vi "Configure Signal (Common).vi"(0 "niUsrpRio Session":T3={"Global Settings Register Bus"=refnum, "Radio 0 Settings Register Bus"=refnum, "Rx NI-USRP session"="", "Tx NI-USRP session"="", "FPGA Interface"=refnum, "RIO Interface Number"=0, "EEPROM Header"={"Checksum"=0, "Product Code"=0, "Hardware Current Version"=0, "Hardware Oldest Compatible Version"=0, "EEPROM Map Current Version"=0, "EEPROM Map Oldest Compatible Version"=0, "User Password"="", "Pointer to Factory Header"=0, "Pointer to User Header"=0, "Recommended Interval"=0, "Number of Reserved Bytes"=9, "Number of Daughterboards"=0, "Daughterboard IDs"=[], "Daughterboard Serial Numbers"=[]}, "Device Data Header"={"Checksum"=0, "Number of Channels"=0, "Number of Gain Settings"=[], "Pointer to Characterization Data"=[], "Number of Reserved Bytes"=27, "Number of Frequencies"=[]}, "EEPROM Characterization Header"={"Checksum"=0, "Date"=timestamp(0 s since 1904-01-01), "Temperature"=0.0, "Misc. Info"="", "Pointer to Device Data Header"=0, "Number of Reserved Bytes"=28}, "Characterization Data"=[], "Characterization Data Valid?"=FALSE, "Radio 1 Settings Register Bus"=refnum, "Radio Settings Bus Semaphore"=refnum} {"Characterization Data"."Frequencies [Hz]" format="%#_6p"; "EEPROM Characterization Header"."Pointer to Device Data Header" format="%x"; "EEPROM Characterization Header"."Checksum" format="%x"; "Device Data Header"."Pointer to Characterization Data" format="%x"; "Device Data Header"."Checksum" format="%x"; "EEPROM Header"."Pointer to User Header" format="%x"; "EEPROM Header"."Pointer to Factory Header" format="%x"; "EEPROM Header"."Product Code" format="%x"; "EEPROM Header"."Checksum" format="%x"}, 1 "scope":string(combo)="rx", 2 "Correct Impairments?":bool=TRUE, 5 "signal parameters":T2={"gain/level"=0.0, "sample rate [S/s]"=10000000.0, "frequency [Hz]"=2450000000.0, "LO frequency [Hz]"=-1.0, "active antenna"="RX1"} {"LO frequency [Hz]" format="%#.3pHz"; "frequency [Hz]" format="%#.3pHz"; "sample rate [S/s]" min=1.0 max=250000000.0 format="%#.3pS/s"}, 7 "Configure Signal Mode":T1, 11 "error in":errorcluster) -> (4 "niUsrpRio Session (out)":T3={"Global Settings Register Bus"=refnum, "Radio 0 Settings Register Bus"=refnum, "Rx NI-USRP session"="", "Tx NI-USRP session"="", "FPGA Interface"=refnum, "RIO Interface Number"=0, "EEPROM Header"={"Checksum"=0, "Product Code"=0, "Hardware Current Version"=0, "Hardware Oldest Compatible Version"=0, "EEPROM Map Current Version"=0, "EEPROM Map Oldest Compatible Version"=0, "User Password"="", "Pointer to Factory Header"=0, "Pointer to User Header"=0, "Recommended Interval"=0, "Number of Reserved Bytes"=9, "Number of Daughterboards"=0, "Daughterboard IDs"=[], "Daughterboard Serial Numbers"=[]}, "Device Data Header"={"Checksum"=0, "Number of Channels"=0, "Number of Gain Settings"=[], "Pointer to Characterization Data"=[], "Number of Reserved Bytes"=27, "Number of Frequencies"=[]}, "EEPROM Characterization Header"={"Checksum"=0, "Date"=timestamp(0 s since 1904-01-01), "Temperature"=0.0, "Misc. Info"="", "Pointer to Device Data Header"=0, "Number of Reserved Bytes"=28}, "Characterization Data"=[], "Characterization Data Valid?"=FALSE, "Radio 1 Settings Register Bus"=refnum, "Radio Settings Bus Semaphore"=refnum} {"Characterization Data"."Frequencies [Hz]" format="%#_6p"; "EEPROM Characterization Header"."Pointer to Device Data Header" format="%x"; "EEPROM Characterization Header"."Checksum" format="%x"; "Device Data Header"."Pointer to Characterization Data" format="%x"; "Device Data Header"."Checksum" format="%x"; "EEPROM Header"."Pointer to User Header" format="%x"; "EEPROM Header"."Pointer to Factory Header" format="%x"; "EEPROM Header"."Product Code" format="%x"; "EEPROM Header"."Checksum" format="%x"}, 6 "coerced signal parameters":T2={"gain/level"=0.0, "sample rate [S/s]"=10000000.0, "frequency [Hz]"=2450000000.0, "LO frequency [Hz]"=-1.0, "active antenna"="RX1"} {"LO frequency [Hz]" format="%#.3pHz"; "frequency [Hz]" format="%#.3pHz"; "sample rate [S/s]" min=1.0 max=250000000.0 format="%#.3pS/s"}, 15 "error out":errorcluster)   [LabVIEW 2013]
doc: "Configures the DSP and signal path for the channel based on the input <B>signal parameters</B>."
uses:
  <instrlib>/niUsrpRio/Config/v1/Host/Public/niUsrpRio Session.ctl
  <instrlib>/_niInstr/Register Bus/v0/Host/Public/Register Bus Session.ctl
  <instrlib>/_niInstr/Register Bus/v0/Host/Private/Session Data.ctl
  <instrlib>/niUsrpRio/Config/v1/Host/Public/EEPROM Header.ctl
  <instrlib>/niUsrpRio/Config/v1/Host/Public/EEPROM Device Data Header.ctl
  <instrlib>/niUsrpRio/Config/v1/Host/Public/EEPROM Characterization Header.ctl
  <instrlib>/niUsrpRio/Config/v1/Host/Public/Characterization Data.ctl
  <instrlib>/niUsrpRio/Config/v1/Host/Public/IQ Imbalance.ctl
  Configure Signal Parameters.ctl
  Configure Signal Mode.ctl
  <instrlib>/_niInstr/DSP/v1/Shared/Public/IQ Impairments.ctl
  Rx FPGA VI Reference.ctl
  Tx FPGA VI Reference.ctl
  <instrlib>/_niInstr/DSP/v1/Shared/Public/IQ Gain.ctl
  <vilib>/rvi/interface/common/niFpgaWaitOnOcc.vi
  <vilib>/Utility/error.llb/Error Cluster From Error Code.vi
  <vilib>/rvi/errors/niLvFpgaAdjustHostInterfaceError.vi
  <vilib>/rvi/interface/nirviReadWriteControl/nirviReadWriteControl.xnode
  <vilib>/ErrorRing/Error Ring.xnode
  NiFpgaLv.dll
  <vilib>/rvi/interface/Simulation/niFpgaSimulationCallBeginRW.vi
  <instrlib>/_niInstr/DSP/v1/Shared/niInstr DSP v1 Shared.lvlib
  <instrlib>/niUsrpRio/Config/v1/Host/niUsrpRio Config v1 Host.lvlib
  <instrlib>/_niInstr/Register Bus/v0/Host/niInstr Register Bus v0 Host.lvlib
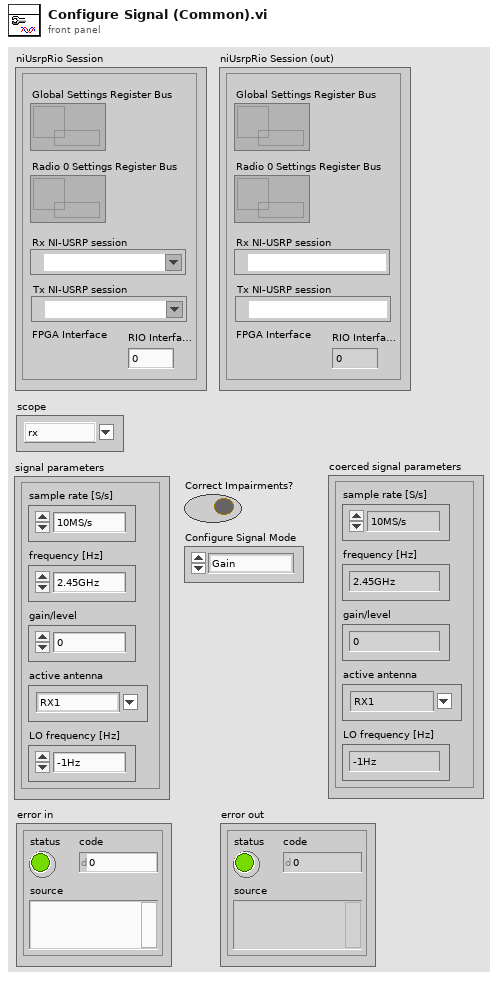
[diagram p1: front panel]
types:
  T1 = typedef "Configure Signal Mode.ctl" = enum16{"Gain", "Level"}
  T2 = typedef "Configure Signal Parameters.ctl" = cluster{"gain/level":dbl, "sample rate [S/s]":dbl, "frequency [Hz]":dbl, "LO frequency [Hz]":dbl, "active antenna":string}
  T3 = typedef "niUsrpRio Config v1 Host.lvlib/niUsrpRio Session.ctl" = cluster{"Global Settings Register Bus":T4, "Radio 0 Settings Register Bus":T4, "Rx NI-USRP session":refnum<k15>, "Tx NI-USRP session":refnum<k15>, "FPGA Interface":refnum<k20>, "RIO Interface Number":u32, "EEPROM Header":T5, "Device Data Header":T6, "EEPROM Characterization Header":T7, "Characterization Data":T8[], "Characterization Data Valid?":bool, "Radio 1 Settings Register Bus":T4, "Radio Settings Bus Semaphore":T10}
  T4 = typedef "niInstr Register Bus v0 Host.lvlib/Register Bus Session.ctl" = refnum<queue>
  T5 = typedef "niUsrpRio Config v1 Host.lvlib/EEPROM Header.ctl" = cluster{"Checksum":u32, "Product Code":u16, "Hardware Current Version":u16, "Hardware Oldest Compatible Version":u16, "EEPROM Map Current Version":u16, "EEPROM Map Oldest Compatible Version":u16, "User Password":string, "Pointer to Factory Header":u32, "Pointer to User Header":u32, "Recommended Interval":u16, "Number of Reserved Bytes":i32, "Number of Daughterboards":u8, "Daughterboard IDs":u16[], "Daughterboard Serial Numbers":string[]}
  T6 = typedef "niUsrpRio Config v1 Host.lvlib/EEPROM Device Data Header.ctl" = cluster{"Checksum":u32, "Number of Channels":u8, "Number of Gain Settings":u16[], "Pointer to Characterization Data":u32[], "Number of Reserved Bytes":i32, "Number of Frequencies":u16[]}
  T7 = typedef "niUsrpRio Config v1 Host.lvlib/EEPROM Characterization Header.ctl" = cluster{"Checksum":u32, "Date":timestamp, "Temperature":sgl, "Misc. Info":string, "Pointer to Device Data Header":u32, "Number of Reserved Bytes":i32}
  T8 = typedef "niUsrpRio Config v1 Host.lvlib/Characterization Data.ctl" = cluster{"Gains[dB]":dbl[], "Frequencies [Hz]":dbl[], "IQ Imbalance Table":T9[], "Measured Gains[dB]":dbl[][]}
  T9 = typedef "niUsrpRio Config v1 Host.lvlib/IQ Imbalance.ctl" = cluster{"Gain Imbalance [linear]":dbl, "Phase Imbalance [radians]":dbl, "Offset":cdb}
  T10 = typedef "Semaphore RefNum" = refnum<k1>
  T11 = typedef "niInstr DSP v1 Shared.lvlib/IQ Impairments.ctl" = cluster{"inline gain I":fxp<+/-,18,1>, "inline gain Q":fxp<+/-,18,1>, "cross gain I":fxp<+/-,18,1>, "cross gain Q":fxp<+/-,18,1>, "pre-gain offset I":fxp<+/-,18,1>, "pre-gain offset Q":fxp<+/-,18,1>, "post-gain offset I":fxp<+/-,18,1>, "post-gain offset Q":fxp<+/-,18,1>}
  T12 = typedef "niUsrpRio Config v1 Host.lvlib/Device Subfunction.ctl" = enum16{"rx", "tx"}
  T13 = typedef "niUsrpRio Config v1 Host.lvlib/RF Channel.ctl" = enum16{"0", "1", "All"}
  T14 = typedef "Rx FPGA VI Reference.ctl" = refnum<k20>
  T15 = typedef "niInstr DSP v1 Shared.lvlib/IQ Gain.ctl" = cluster{"gain I":fxp<+/-,24,3>, "gain Q":fxp<+/-,24,3>}
  T16 = typedef "Tx FPGA VI Reference.ctl" = refnum<k20>
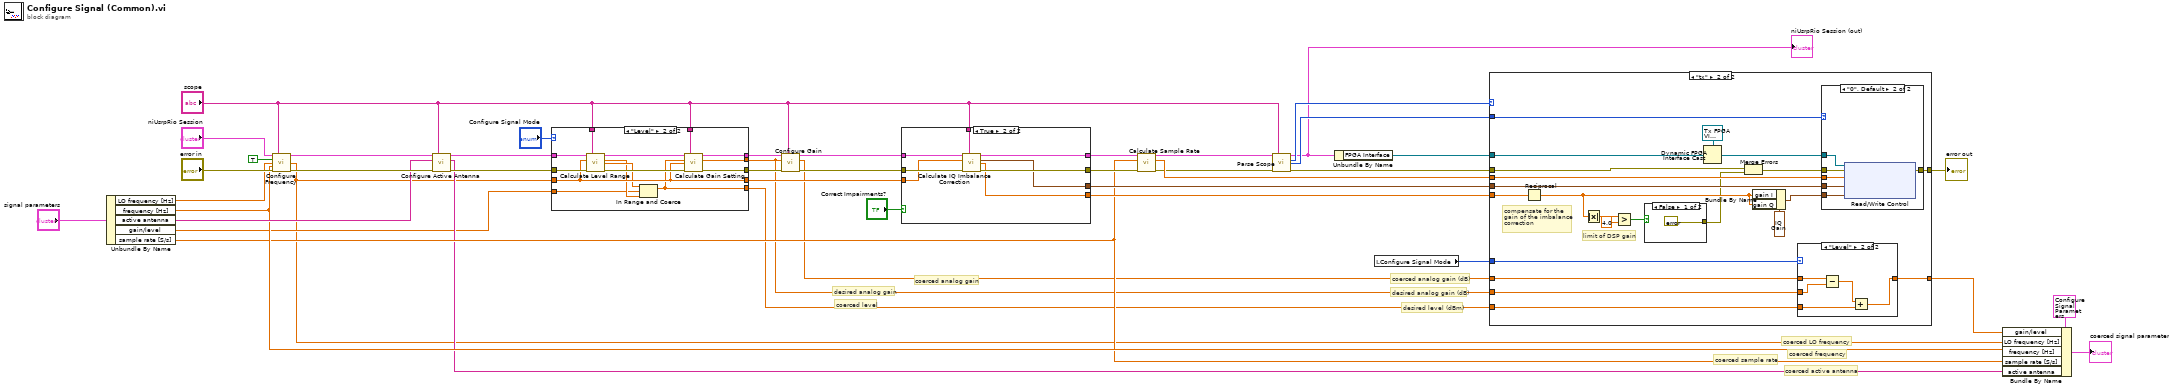
[diagram p0: block diagram]
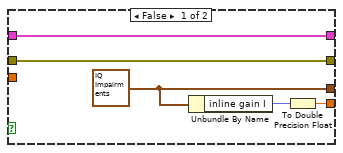
[diagram p3: hidden frame]
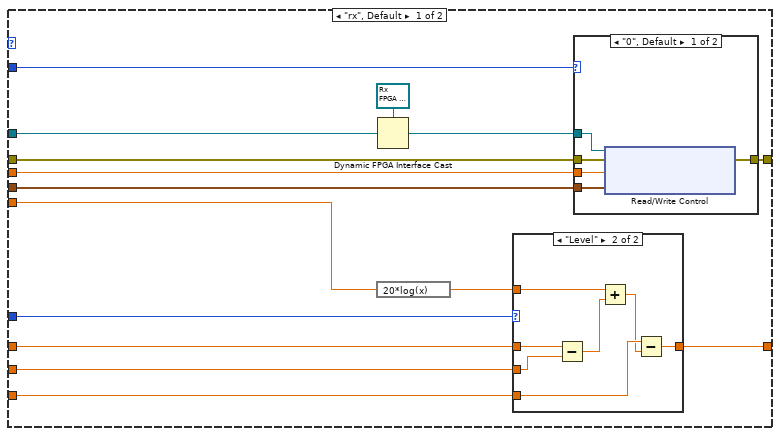
[diagram p4: hidden frame]
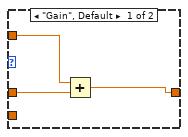
[diagram p5: hidden frame]
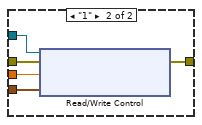
[diagram p6: hidden frame]
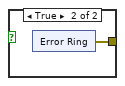
[diagram p7: hidden frame]
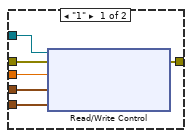
[diagram p9: hidden frame]
diagram:
  # "coerced level"
  # "desired level (dBm)"
  # "desired analog gain"
  # "desired analog gain (dB)"
  # "coerced analog gain (dB)"
  # "coerced analog gain"
  # "coerced active antenna"
  # "coerced sample rate"
  # "coerced frequency"
  # "coerced LO frequency"
  n1 = Unbundle By Name("signal parameters") -> ("LO frequency [Hz]"=w24:dbl, "frequency [Hz]"=w13:dbl, "active antenna"=w23:string, "gain/level"=w6:dbl, "sample rate [S/s]"=w12:dbl)
  n2 = call "Configure Frequency.vi"("niUsrpRio Session"="niUsrpRio Session", "scope"="scope", "wait for lo to lock"=TRUE, "lo frequency"=w24, "frequency"=w13, "error in"="error in") -> ("niUsrpRio Session (out)"=w32:T3, "coerced lo frequency"=w4:dbl, "error out"=w31:errorcluster)  [unwired: 7 in]
  n3 = call <instrlib>:"Configure Active Antenna.vi"("niUsrpRio session"=w32, "scope"="scope", "active antenna"=w23, "Error In"=w31) -> ("niUsrpRio session (out)"=w21:T3, "coerced active antenna"=w11:string, "Error Out"=w20:errorcluster)  [unwired: 9 in]
  n4 = case shown="\"Level\"" "Configure Signal Mode" {
    tunnel: w21 -> [w46 w51]
    tunnel: w20 -> [w45 w60]
    tunnel: w6 -> [w44 w52]
    tunnel: "scope" -> [_ w57]
    tunnel: [w46 w56] -> w17
    tunnel: w4 -> [w47 w58]
    tunnel: [w47 w58] -> w19
    tunnel: [w45 w61] -> w18
    tunnel: [w44 w55] -> w7
    tunnel: "scope" -> [_ w49]
    tunnel: [w44 w48] -> w1
    frame "Gain", Default {
    }
    frame "Level" {
      n5 = call <instrlib>:"Calculate Level Range.vi"("niUsrpRio Session"=w51, "scope"=w49, "frequency"=w58, "error in"=w60) -> ("niUsrpRio Session (out)"=w50:T3, "Min Level"=w53:dbl, "Max Level"=w54:dbl, "error out"=w59:errorcluster)  [unwired: 8 in]
      n6 = In Range and Coerce(upper limit=w54, x=w52, lower limit=w53) -> (coerced(x)=w48:dbl)  [unwired: 1 out]
      n7 = call <instrlib>:"Calculate Gain Setting.vi"("niUsrpRio Session"=w50, "scope"=w57, "level"=w48, "frequency"=w58, "error in"=w59) -> ("niUsrpRio Session (out)"=w56:T3, "gain"=w55:dbl, "error out"=w61:errorcluster)  [unwired: 8 in]
    }
  }
  n8 = call <instrlib>:"Configure Gain.vi"("niUsrpRio session"=w17, "scope"="scope", "gain"=w7, "Error In"=w18) -> ("niUsrpRio session (out)"=w16:T3, "coerced gain"=w8:dbl, "Error Out"=w15:errorcluster)  [unwired: 9 in]
  n9 = case shown="True" "Correct Impairments?" {
    tunnel: w15 -> [w65 w73]
    tunnel: w16 -> [w66 w74]
    tunnel: "scope" -> [_ w72]
    tunnel: [w66 w71] -> w27
    tunnel: [w65 w70] -> w26
    tunnel: [w62 w69] -> w29
    tunnel: [w63 w67] -> w28
    tunnel: w19 -> [_ w68]
    frame False {
      w62 = T11 {"inline gain I"=0.9999923706054688, "inline gain Q"=0.9999923706054688, "cross gain I"=0.0, "cross gain Q"=0.0, "pre-gain offset I"=0.0, "pre-gain offset Q"=0.0, "post-gain offset I"=0.0, "post-gain offset Q"=0.0} ("impairment control")
      n10 = Unbundle By Name(w62) -> ("inline gain I"=w64:fxp<+/-,18,1>)
      n11 = To Double Precision Float(number=w64) -> (double precision float=w63:dbl)
    }
    frame True {
      n12 = call <instrlib>:"Calculate IQ Imbalance Correction.vi"("niUsrpRio Session"=w74, "scope"=w72, "frequency"=w68, "error in"=w73) -> ("niUsrpRio Session (out)"=w71:T3, "IQ imbalance correction"=w69:T11, "correction gain"=w67:dbl, "error out"=w70:errorcluster)  [unwired: 8 in]
    }
  }
  n13 = call "Calculate Sample Rate.vi"("niUsrpRio Session"=w27, "sample rate [S/s]"=w12, "error in"=w26) -> ("niUsrpRio Session (out)"=w39:T3, "sample rate [ratio]"=w43:dbl, "error out"=w38:errorcluster)  [unwired: 10 in]
  n14 = call <instrlib>:"Parse Scope.vi"("niUsrpRio Session"=w39, "scope"="scope", "Error In"=w38) -> ("niUsrpRio Session (out)"=w35:T3, "Device Subfunction"=w37:T12, "Device Subfunction Channel"=w36:T13, "Error Out"=w34:errorcluster)  [unwired: 4 in, 5 out]
  "niUsrpRio Session (out)" <- w35
  n15 = Unbundle By Name(w35) -> ("FPGA Interface"=w33:refnum<k20>)
  n16 = local read "Configure Signal Mode"() -> (w9:T1)
  n17 = case shown="\"tx\"" w37 {
    tunnel: w43 -> [w89 w131]
    tunnel: w33 -> [w88 w130]
    tunnel: [w87 w129] -> w42
    tunnel: w34 -> [w86 w128]
    tunnel: w29 -> [w83 w125]
    tunnel: w36 -> [w82 w124]
    tunnel: w28 -> [w81 w122]
    tunnel: w9 -> [w79 w120]
    tunnel: w8 -> [w80 w119]
    tunnel: [w77 w118] -> w5
    tunnel: w7 -> [w75 w117]
    tunnel: w1 -> [w76 w116]
    frame "rx", Default {
      n18 = expression code="20*log(x)"(w81) -> (w78:dbl)
      n19 = Dynamic FPGA Interface Cast(Session In=T14 refnum ("FPGA VI Reference Out"), Type=w88) -> (Session Out=w84:T14)
      n20 = case shown="\"Level\"" w79 {
        tunnel: w80 -> [w91 w99]
        tunnel: [w90 w93] -> w77
        tunnel: w75 -> [_ w98]
        tunnel: w76 -> [_ w95]
        tunnel: w78 -> [w92 w97]
        frame "Gain", Default {
          n21 = Add(x=w92, y=w91) -> (x+y=w90:dbl)
        }
        frame "Level" {
          n22 = Subtract(x=w99, y=w98) -> (x-y=w96:dbl)
          n23 = Add(x=w97, y=w96) -> (x+y=w94:dbl)
          n24 = Subtract(x=w95, y=w94) -> (x-y=w93:dbl)
        }
      }
      n25 = case shown="\"0\", Default" w82 {
        tunnel: w89 -> [w102 w109]
        tunnel: [w100 w108] -> w87
        tunnel: w86 -> [w104 w107]
        tunnel: w84 -> [w103 w106]
        tunnel: w83 -> [w101 w105]
        frame "0", Default {
          n26 = xnode "Read/Write Control"("FPGA VI Reference In"=w103, "error in"=w104, "rx.output sample rate"=w102, "rx 0.impairments"=w101) -> ("error out"=w100:errorcluster)  [unwired: 1 out]
        }
        frame "1" {
          n27 = xnode "Read/Write Control"("FPGA VI Reference In"=w106, "error in"=w107, "rx.output sample rate"=w109, "rx 1.impairments"=w105) -> ("error out"=w108:errorcluster)  [unwired: 1 out]
        }
      }
    }
    frame "tx" {
      # "limit of DSP gain"
      # "compensate for the\ngain of the imbalance\ncorrection"
      n28 = Reciprocal(x=w122) -> (1/x=w114:dbl)
      n29 = Absolute Value(x=w114) -> (abs(x)=w112:dbl)
      n30 = Greater?(x=w112, y=4.0) -> (0:w115:bool)
      n31 = case shown="False" w115 {
        tunnel: [errorcluster {"status"=FALSE, "code"=0, "source"=""} ("error constant") w133] -> w110
        frame False {
        }
        frame True {
          n32 = xnode "Error Ring"() -> ("error out"=w133:errorcluster)
        }
      }
      n33 = Dynamic FPGA Interface Cast(Session In=T16 refnum ("FPGA VI Reference Out"), Type=w130) -> (Session Out=w126:T16)
      n34 = Merge Errors(w128, w110) -> (w111:errorcluster)
      n35 = Bundle By Name(cluster=T15 {"gain I"=1.0, "gain Q"=1.0} ("gain"), "gain I"=w114, "gain Q"=w114) -> (w121:T15)
      n36 = case shown="\"Level\"" w120 {
        tunnel: w119 -> [w139 w144]
        tunnel: [w139 w140] -> w118
        tunnel: w117 -> [_ w143]
        tunnel: w116 -> [_ w142]
        frame "Gain", Default {
        }
        frame "Level" {
          n37 = Subtract(x=w144, y=w143) -> (x-y=w141:dbl)
          n38 = Add(x=w141, y=w142) -> (x+y=w140:dbl)
        }
      }
      n39 = case shown="\"0\", Default" w124 {
        tunnel: w131 -> [w150 w156]
        tunnel: [w149 w155] -> w129
        tunnel: w111 -> [w148 w154]
        tunnel: w126 -> [w147 w153]
        tunnel: w125 -> [w146 w152]
        tunnel: w121 -> [w145 w151]
        frame "1" {
          n40 = xnode "Read/Write Control"("FPGA VI Reference In"=w147, "error in"=w148, "tx.input sample rate"=w150, "tx 1.impairments"=w146, "tx 1.gain"=w145) -> ("error out"=w149:errorcluster)  [unwired: 1 out]
        }
        frame "0", Default {
          n41 = xnode "Read/Write Control"("FPGA VI Reference In"=w153, "error in"=w154, "tx.input sample rate"=w156, "tx 0.impairments"=w152, "tx 0.gain"=w151) -> ("error out"=w155:errorcluster)  [unwired: 1 out]
        }
      }
    }
  }
  "error out" <- w42
  n42 = Bundle By Name(cluster=T2 {"gain/level"=0.0, "sample rate [S/s]"=10000000.0, "frequency [Hz]"=2450000000.0, "LO frequency [Hz]"=-1.0, "active antenna"="RX1"} ("coerced signal parameters"), "gain/level"=w5, "LO frequency [Hz]"=w4, "frequency [Hz]"=w13, "sample rate [S/s]"=w12, "active antenna"=w11) -> (→"coerced signal parameters":T2)
